vi "check for new error.vi"(7 "Send Stop on Fail (F)":bool, 8 "Error to Process":errorcluster, 11 "Template in":refnum<class "Template.lvclass">) -> ()   [LabVIEW 2020, in "Template.lvlib" / "Template.lvclass"]
uses:
  Template.lvclass
  C:/Program Files/National Instruments/LabVIEW 2020/vi.lib/ActorFramework/Actor/Actor.lvclass
  <vilib>/ActorFramework/Actor/Actor.lvclass/Actor.ctl
  <vilib>/ActorFramework/Message Enqueuer/Message Enqueuer.lvclass/Message Enqueuer.ctl
  <vilib>/ActorFramework/Message Enqueuer/Message Priority.ctl
  Template Messages/fire error object Msg/fire error object Msg.lvclass/fire error object Msg.ctl
  <vilib>/ActorFramework/Stop Msg/Stop Msg.lvclass/Stop Msg.ctl
  <vilib>/ActorFramework/Message Enqueuer/Enqueue.vi
  <vilib>/ActorFramework/Message Enqueuer/Enqueue Critical.vi
  <vilib>/ActorFramework/Message Enqueuer/Init from Existing Queue.vi
  Template Messages/fire error object Msg/fire error object Msg.lvclass
  C:/Program Files/National Instruments/LabVIEW 2020/vi.lib/ActorFramework/Message/Message.lvclass
  <vilib>/ActorFramework/Stop Msg/Stop Msg.lvclass
  <vilib>/ActorFramework/Message Priority Queue/Priority Enqueue.vi
  <vilib>/ActorFramework/Message Enqueuer/Message Enqueuer.lvclass
  interfaces/Error Interface/Error/Error.lvclass
  <vilib>/ActorFramework/Actor/Actor.lvclass
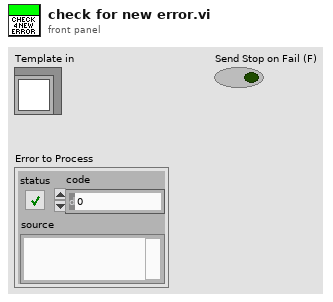
[diagram p1: front panel]
types:
  T1 = typedef "Actor Framework.lvlib/Message Enqueuer.lvclass/Message Priority.ctl" = enum16{"Low", "Normal", "High"}
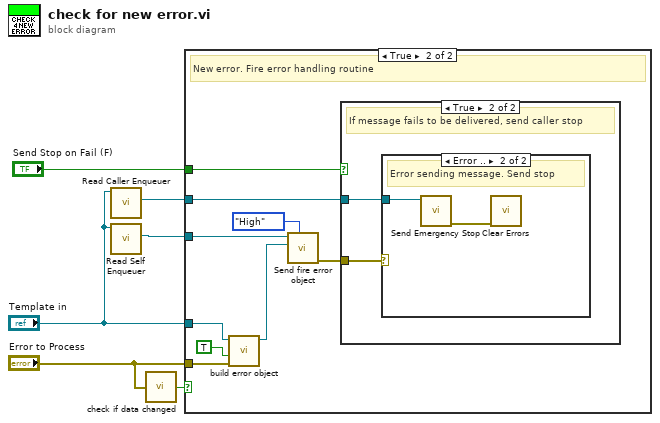
[diagram p0: block diagram]
diagram:
  n1 = call <vilib>:"Read Caller Enqueuer.vi"("Actor"="Template in") -> ("Caller Enqueuer"=w1:refnum<class "Message Enqueuer.lvclass">)  [unwired: 10 in]
  n2 = call <vilib>:"Read Self Enqueuer.vi"("Actor"="Template in") -> ("Self Enqueuer"=w3:refnum<class "Message Enqueuer.lvclass">)  [unwired: 10 in]
  n3 = call "check if data changed.vi"("Data"="Error to Process") -> ("Data Changed?"=w5:bool)  [unwired: 4 in]
  n4 = case shown="True" w5 {
    tunnel: "Template in" -> [_ w15]
    tunnel: "Error to Process" -> [_ w12]
    tunnel: w3 -> [_ w9]
    tunnel: "Send Stop on Fail (F)" -> [_ w8]
    tunnel: w1 -> [_ w7]
    frame False {
      # "Not a new error."
    }
    frame True {
      # "New error. Fire error handling routine"
      n5 = call "build error object.vi"("Error to Process"=w12, "Report Error (F)"=TRUE, "Error Location"=w15) -> ("Error object"=w14:refnum<class>)  [unwired: 8 in]
      n6 = call "Send fire error object.vi"("Message Priority (Normal)"=Message_Priority."High", "Error in"=w14, "Message Enqueuer"=w9) -> ("error out"=w10:errorcluster)  [unwired: 7 in, 1 out]
      n7 = case shown="True" w8 {
        tunnel: w10 -> [_ w17]
        tunnel: w7 -> [_ w16]
        frame False {
        }
        frame True {
          # "If message fails to be delivered, send caller stop"
          n8 = case shown="Error .." w17 {
            tunnel: w16 -> [_ w18]
            frame No Error {
              # "Message sent. Do Nothing"
            }
            frame Error {
              # "Error sending message. Send stop"
              n9 = call <vilib>:"Send Emergency Stop.vi"("Message Enqueuer"=w18) -> ("error out"=w19:errorcluster)  [unwired: 10 in]
              n10 = call <vilib>:"Clear Errors.vi"("error in (no error)"=w19) -> ()  [unwired: 5 in, 2 out]
            }
          }
        }
      }
    }
  }
